vi "Acoustic modem TCPIP.vi"(2 "strings num":i32, 6 "Enum":T1(ring)=enum."bitrate", 7 "lOPP COUNT":i32, 8 "error in (no error)":errorcluster, 10 "Read/Write":bool, 11 "Cluster":T2) -> (0 "error out":errorcluster, 4 "Data Tx/Rx":string, 5 "Data out":string)   [LabVIEW 2021]
uses:
  183c8938-68d7-426e-a12b-0680b4555289.vi
panel:
  in  "error out 2":errorcluster
  out "x-y":u32
  out "WRITE BUTTON":bool
  in  "Write Power Status":bool
  out "match substring":string
  out "Modem Ready Status":bool
  out "length":i32
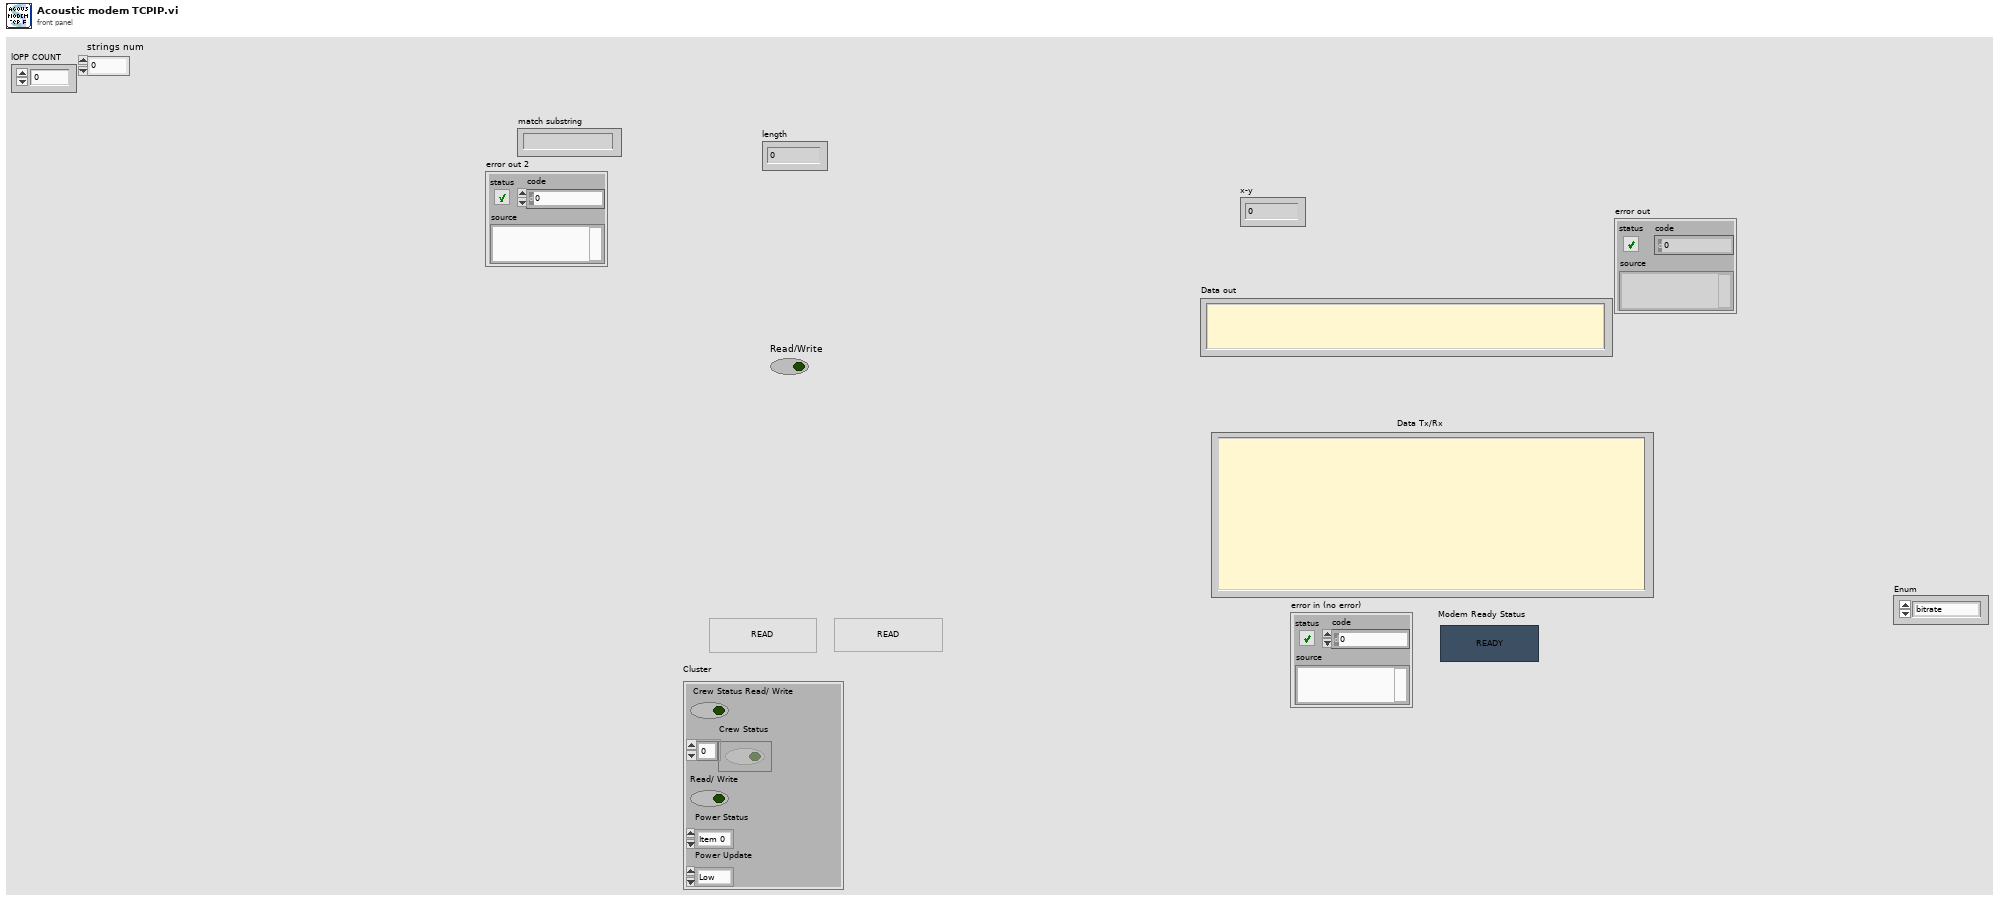
[diagram p1: front panel]
types:
  T1 = enum16{"TCPIP acoustic stop", "read write state", "command mode", "Disable Extended Notification", "bitrate", "initialization", "Int Power Status"}
  T2 = cluster{" Crew Status Read/ Write":bool, "Crew Status":bool[], "Read/ Write":bool, "Power Status":enum32{"Item 0", "Item 1", "Item 2", "Item 3"}, "Power Update":enum16{"Low", "Medium", "High", "Very High"}}
  T3 = cluster{"navigation":string, "HSSS":string, "P1":string, "P2":string}
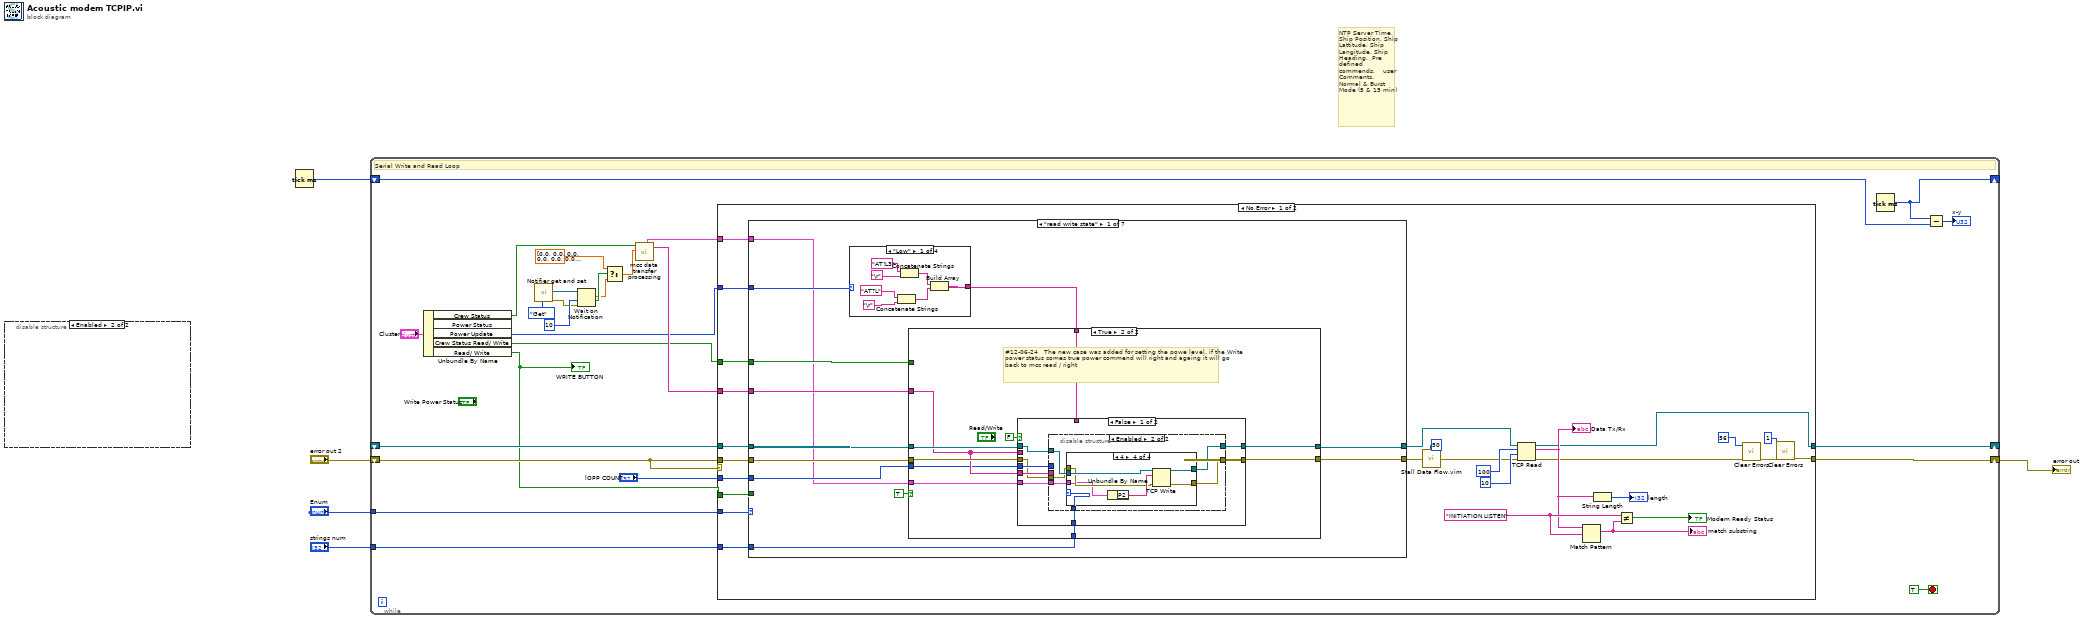
[diagram p0: block diagram]
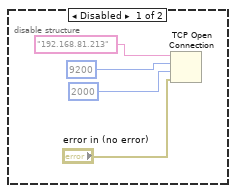
[diagram p2: hidden frame]
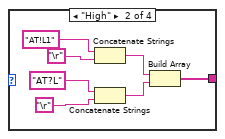
[diagram p3: hidden frame]
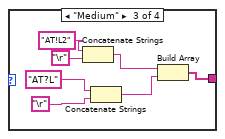
[diagram p4: hidden frame]
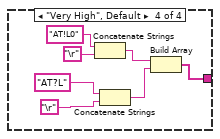
[diagram p5: hidden frame]
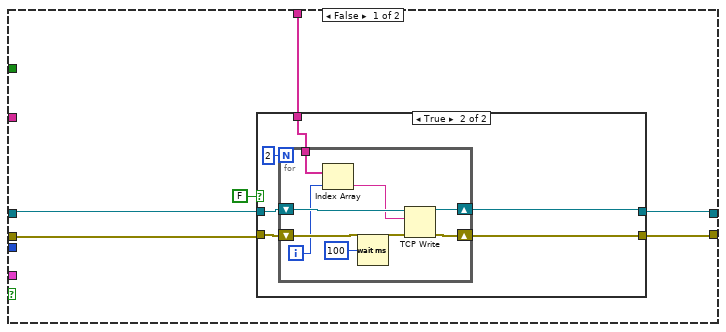
[diagram p6: hidden frame]
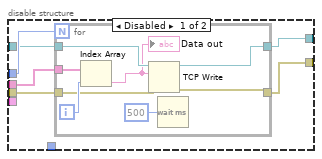
[diagram p8: hidden frame]
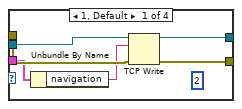
[diagram p9: hidden frame]
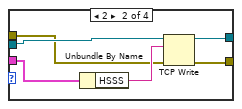
[diagram p10: hidden frame]
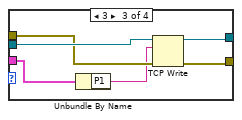
[diagram p11: hidden frame]
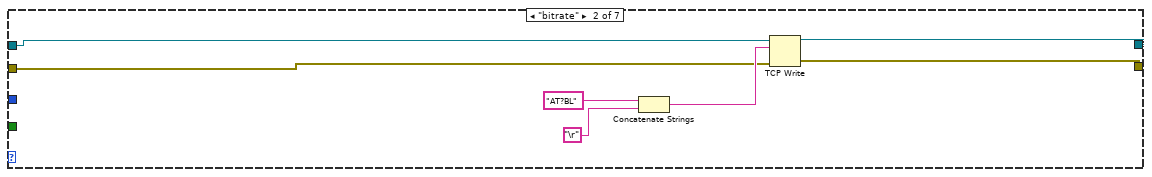
[diagram p13: hidden frame]
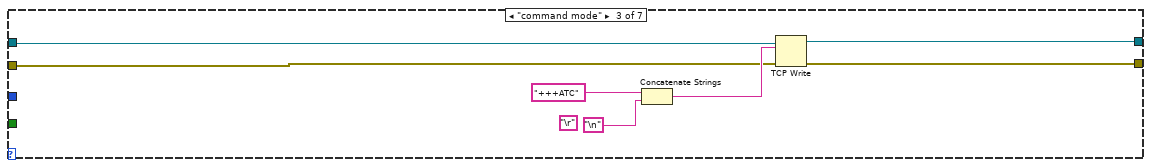
[diagram p14: hidden frame]
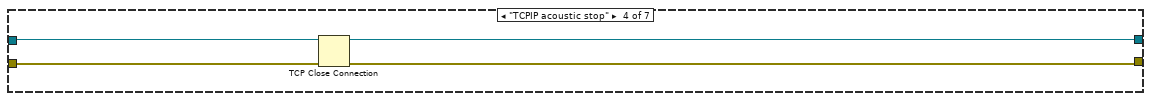
[diagram p15: hidden frame]
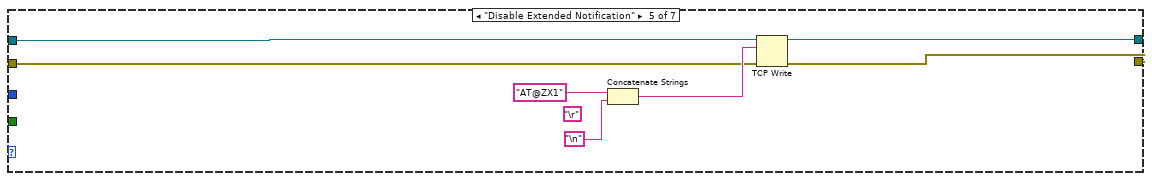
[diagram p16: hidden frame]
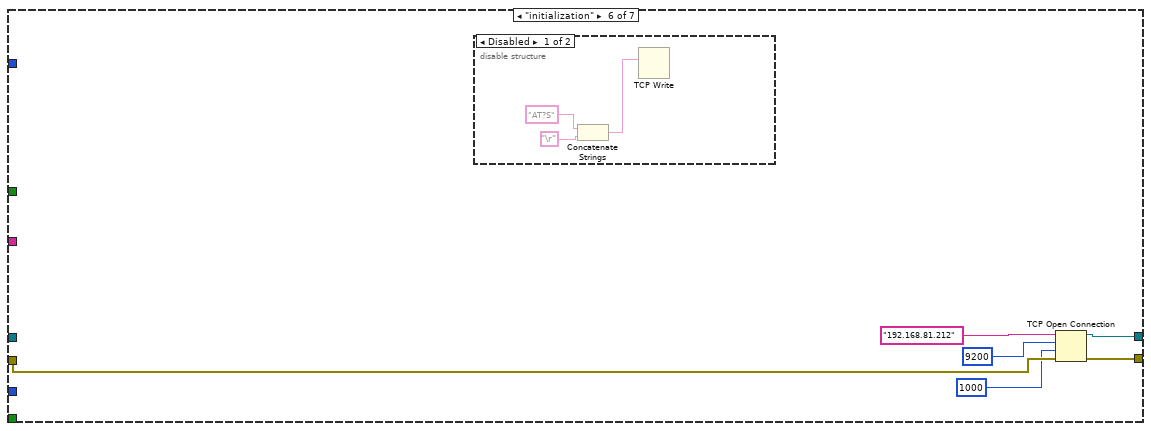
[diagram p17: hidden frame]
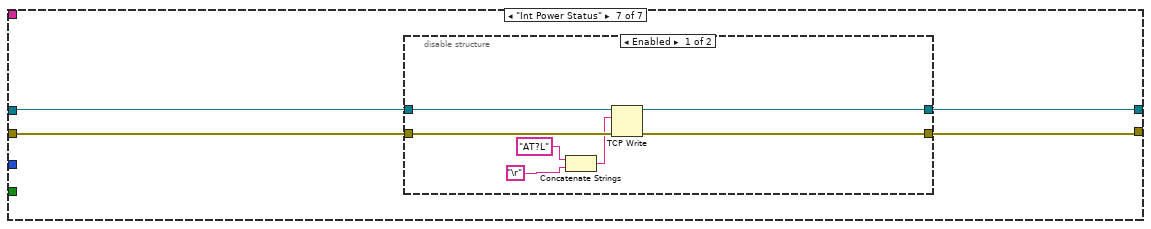
[diagram p19: hidden frame]
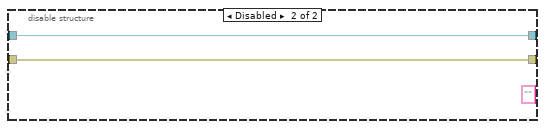
[diagram p20: hidden frame]
diagram:
  # "NTP Server Time, Ship Position, Ship Lattitude, Ship Langitude, Ship Heading,  Pre defined commends,    user Comments.  Normal & Burst Mode (5 & 15 min)"
  n1 = disable-structure shown="Enabled" {
    frame Disabled {
      n2 = TCP Open Connection(address="192.168.81.213", remote port or service name=u16 9200, timeout ms (60000)=2000, error in (no error)="error in (no error)") -> ()  [unwired: 1 in, 2 out]
    }
    frame Enabled {
    }
  }
  n3 = Tick Count (ms)() -> (millisecond timer value=w4:u32)
  n4 = while {
    shift-right: [w32] -> _
    shift-left: _ -> [w35]
    shift-right: [w31] -> w3
    shift-left: "error out 2" -> [w34]
    tunnel: "Enum" -> [w33]
    shift-right: [w14] -> _
    shift-left: w4 -> [w13]
    tunnel: "strings num" -> [w12]
    stop <- TRUE stop-if-true
    # "Serial Write and Read Loop"
    n5 = Unbundle By Name("Cluster") -> ("Crew Status"=w27:bool[], "Power Update"=w26:enum16{"Low", "Medium", "High", "Very High"}, "Crew Status Read/ Write"=w25:bool, "Read/ Write"=w24:bool)  [unwired: 1 out]
    "WRITE BUTTON" <- w24
    n6 = call "Notifier get and set.vi"("Operation"=enum16{"Init", "Get", "Set"}."Get") -> ("error out"=w18:errorcluster, "notifier out"=w21:refnum<notifier>)  [unwired: 9 in]
    n7 = Wait on Notification(notifier=w21, timeout in ms (-1)=10, error in (no error)=w18) -> (notification=w16:dbl[], timed out?=w17:bool)  [unwired: 1 in, 2 out]
    n8 = Select(t=dbl[] [0.0, 0.0, 0.0, 0.0, 0.0, 0.0, 0.0, 0.0, 0.0, 0.0, 0.0, 0.0, 0.0, 0.0, 0.0, 0.0, 0.0, 0.0, 0.0, 0.0, 0.0, 0.0, 0.0, 0.0, 0.0, 0.0, 0.0, 0.0, 0.0, 0.0, 0.0, 0.0, 0.0, 0.0, 0.0, 0.0, 0.0, 0.0, 0.0, 0.0, 0.0, 0.0, 0.0, 0.0, 0.0, 0.0, 0.0, 0.0, 0.0, 0.0, 0.0], s=w17, f=w16) -> (s? t:f=w22:dbl[])
    n9 = call "mcc data transfer processing.vi"("s? t:f"=w22, "Crew Status"=w27) -> ("output cluster"=w11:T3, "appended array"=w30:string[])  [unwired: 3 in, 4 out]
    n10 = case shown="No Error" w34 {
      selector: w34 -> [_ w238]
      tunnel: w35 -> [w62 _]
      tunnel: w34 -> [w61 _]
      tunnel: [w39 w242] -> w32
      tunnel: [w40 w241] -> w31
      tunnel: w24 -> [w57 _]
      tunnel: w33 -> [w54 _]
      tunnel: w30 -> [w53 _]
      tunnel: w25 -> [w51 _]
      tunnel: w26 -> [w49 _]
      tunnel: "lOPP COUNT" -> [w48 _]
      tunnel: w12 -> [w37 _]
      tunnel: w11 -> [w36 _]
      frame No Error {
        w60 = "INITIATION LISTEN"
        n11 = case shown="\"read write state\"" w54 {
          tunnel: w62 -> [w74 w189 w200 w206 w211 _ w225]
          tunnel: w61 -> [w73 w190 w199 w205 w210 w217 w226]
          tunnel: [w72 w191 w198 w204 w209 w215 w224] -> w45
          tunnel: [w71 w192 w197 w203 w208 w214 w223] -> w52
          tunnel: w57 -> [_ _ _ _ _ _ _]
          tunnel: w53 -> [w70 _ _ _ _ _ _]
          tunnel: w51 -> [w68 _ _ _ _ _ _]
          tunnel: w49 -> [w67 _ _ _ _ _ _]
          tunnel: w48 -> [w66 _ _ _ _ _ _]
          tunnel: w37 -> [w64 _ _ _ _ _ _]
          tunnel: w36 -> [w63 _ _ _ _ _ _]
          frame "read write state" {
            n12 = case shown="\"Low\"" w67 {
              tunnel: [w75 w84 w91 w96] -> w69
              frame "Low" {
                n13 = Concatenate Strings("AT?L" ("write buffer"), "\r") -> (w76:string)
                n14 = Concatenate Strings("AT!L3" ("string"), "\r") -> (w77:string)
                n15 = Build Array(w77, w76) -> (w75:string[])
              }
              frame "High" {
                n16 = Concatenate Strings("AT!L1" ("string"), "\r") -> (w83:string)
                n17 = Concatenate Strings("AT?L" ("write buffer"), "\r") -> (w82:string)
                n18 = Build Array(w83, w82) -> (w84:string[])
              }
              frame "Medium" {
                n19 = Concatenate Strings("AT!L2" ("string"), "\r") -> (w90:string)
                n20 = Concatenate Strings("AT?L" ("write buffer"), "\r") -> (w89:string)
                n21 = Build Array(w90, w89) -> (w91:string[])
              }
              frame "Very High", Default {
                n22 = Concatenate Strings("AT!L0" ("string"), "\r") -> (w98:string)
                n23 = Concatenate Strings("AT?L" ("write buffer"), "\r") -> (w97:string)
                n24 = Build Array(w98, w97) -> (w96:string[])
              }
            }
            n25 = case shown="True" TRUE {
              tunnel: w74 -> [w106 w134]
              tunnel: w73 -> [w108 w133]
              tunnel: [w105 w132] -> w72
              tunnel: [w107 w131] -> w71
              tunnel: w70 -> [_ w129]
              tunnel: w69 -> [w104 w130]
              tunnel: w68 -> [_ _]
              tunnel: w66 -> [_ w128]
              tunnel: w64 -> [_ w127]
              tunnel: w63 -> [_ w126]
              frame False {
                n26 = case shown="True" FALSE {
                  tunnel: w106 -> [w110 w115]
                  tunnel: w108 -> [w109 w116]
                  tunnel: [w110 w112] -> w105
                  tunnel: [w109 w111] -> w107
                  tunnel: w104 -> [_ w114]
                  frame False {
                  }
                  frame True {
                    n27 = for {
                      N: 2 -> [_]
                      tunnel: w114 -> [w119]
                      shift-right: [w121] -> w111
                      shift-left: w116 -> [w124]
                      shift-right: [w122] -> w112
                      shift-left: w115 -> [w123]
                      i -> [w120]
                      n28 = Index Array(array=w119, index=w120) -> (element=w118:string)
                      n29 = Wait (ms)(milliseconds to wait=u32 100) -> ()  [unwired: 1 out]
                      n30 = TCP Write(connection ID=w123, data in=w118, error in (no error)=w124) -> (connection ID out=w122:refnum<k5>, error out=w121:errorcluster)  [unwired: 1 in, 1 out]
                    }
                  }
                }
              }
              frame True {
                # "#12-06-24   The new case was added for setting the powe level. if the Write power status comes true power commend will right and againg it will go back to mcc read / right"
                n31 = case shown="False" FALSE {
                  tunnel: w134 -> [w140 w188]
                  tunnel: w133 -> [w139 w187]
                  tunnel: [w138 w188] -> w132
                  tunnel: [w137 w187] -> w131
                  tunnel: w129 -> [_ _]
                  tunnel: w130 -> [_ _]
                  tunnel: w129 -> [w142 _]
                  tunnel: w128 -> [w141 _]
                  tunnel: w127 -> [w136 _]
                  tunnel: w126 -> [w135 _]
                  frame False {
                    n32 = disable-structure shown="Enabled" {
                      disable-tunnel: w142 -> [w148 _]
                      disable-tunnel: w141 -> [w147 _]
                      disable-tunnel: w140 -> [w146 w160]
                      disable-tunnel: w139 -> [w145 w159]
                      disable-tunnel: [w144 w158] -> w138
                      disable-tunnel: [w143 w157] -> w137
                      disable-tunnel: w136 -> [_ w162]
                      disable-tunnel: w135 -> [_ w161]
                      frame Disabled {
                        n33 = for {
                          N: w147 -> [_]
                          tunnel: w148 -> [w156]
                          tunnel: w146 -> [w154]
                          tunnel: [w152] -> w144
                          tunnel: w145 -> [w153]
                          tunnel: [w151] -> w143
                          i -> [w155]
                          n34 = Index Array(array=w156, index=w155) -> (element=w150:string)
                          "Data out" <- w150
                          n35 = TCP Write(connection ID=w154, data in=w150, error in (no error)=w153) -> (connection ID out=w152:refnum<k5>, error out=w151:errorcluster)  [unwired: 1 in, 1 out]
                          n36 = Wait (ms)(milliseconds to wait=u32 500) -> ()  [unwired: 1 out]
                        }
                      }
                      frame Enabled {
                        n37 = case shown="4" w162 {
                          tunnel: w161 -> [w166 w173 w175 w181]
                          tunnel: w160 -> [w168 w172 w178 w183]
                          tunnel: w159 -> [w167 w171 w177 w182]
                          tunnel: [w164 w170 w180 w184] -> w158
                          tunnel: [w163 w169 w179 w185] -> w157
                          frame 1, Default {
                            (unwired) 2
                            n38 = Unbundle By Name(w166) -> ("navigation"=w165:string)
                            n39 = TCP Write(connection ID=w168, data in=w165, error in (no error)=w167) -> (connection ID out=w164:refnum<k5>, error out=w163:errorcluster)  [unwired: 1 in, 1 out]
                          }
                          frame 2 {
                            n40 = Unbundle By Name(w173) -> ("HSSS"=w174:string)
                            n41 = TCP Write(connection ID=w172, data in=w174, error in (no error)=w171) -> (connection ID out=w170:refnum<k5>, error out=w169:errorcluster)  [unwired: 1 in, 1 out]
                          }
                          frame 3 {
                            n42 = Unbundle By Name(w175) -> ("P1"=w176:string)
                            n43 = TCP Write(connection ID=w178, data in=w176, error in (no error)=w177) -> (connection ID out=w180:refnum<k5>, error out=w179:errorcluster)  [unwired: 1 in, 1 out]
                          }
                          frame 4 {
                            n44 = Unbundle By Name(w181) -> ("P2"=w186:string)
                            n45 = TCP Write(connection ID=w183, data in=w186, error in (no error)=w182) -> (connection ID out=w184:refnum<k5>, error out=w185:errorcluster)  [unwired: 1 in, 1 out]
                          }
                        }
                      }
                    }
                  }
                  frame True {
                  }
                }
              }
            }
          }
          frame "bitrate" {
            n46 = Concatenate Strings("AT?BL" ("string"), "\r") -> (w195:string)
            n47 = TCP Write(connection ID=w189, data in=w195, error in (no error)=w190) -> (connection ID out=w191:refnum<k5>, error out=w192:errorcluster)  [unwired: 1 in, 1 out]
          }
          frame "command mode" {
            (unwired) "\r"
            n48 = Concatenate Strings("+++ATC" ("string"), "\n") -> (w201:string)
            n49 = TCP Write(connection ID=w200, data in=w201, error in (no error)=w199) -> (connection ID out=w198:refnum<k5>, error out=w197:errorcluster)  [unwired: 1 in, 1 out]
          }
          frame "TCPIP acoustic stop" {
            n50 = TCP Close Connection(connection ID=w206, error in (no error)=w205) -> (connection ID out=w204:refnum<k5>, error out=w203:errorcluster)  [unwired: 1 in]
          }
          frame "Disable Extended Notification" {
            (unwired) "\r"
            n51 = Concatenate Strings("AT@ZX1" ("string"), "\n") -> (w213:string)
            n52 = TCP Write(connection ID=w211, data in=w213, error in (no error)=w210) -> (connection ID out=w209:refnum<k5>, error out=w208:errorcluster)  [unwired: 1 in, 1 out]
          }
          frame "initialization" {
            n53 = disable-structure shown="Disabled" {
              frame Disabled {
                n54 = Concatenate Strings("AT?S" ("string"), "\r") -> (w222:string)
                n55 = TCP Write(data in=w222) -> ()  [unwired: 3 in, 3 out]
              }
              frame Enabled {
              }
            }
            n56 = TCP Open Connection(address="192.168.81.212", remote port or service name=u16 9200, timeout ms (60000)=1000, error in (no error)=w217) -> (connection ID=w215:refnum<k5>, error out=w214:errorcluster)  [unwired: 1 in]
          }
          frame "Int Power Status" {
            n57 = disable-structure shown="Enabled" {
              disable-tunnel: w226 -> [w233 w235]
              disable-tunnel: w225 -> [w232 w236]
              disable-tunnel: [w227 w236] -> w224
              disable-tunnel: [w228 w235] -> w223
              frame Enabled {
                n58 = Concatenate Strings("AT?L" ("write buffer"), "\r") -> (w230:string)
                n59 = TCP Write(connection ID=w232, data in=w230, error in (no error)=w233) -> (connection ID out=w227:refnum<k5>, error out=w228:errorcluster)  [unwired: 1 in, 1 out]
              }
              frame Disabled {
                w234 = "" ("read buffer")
              }
            }
          }
        }
        n60 = call "Stall Data Flow.vim"("value in"=w52, "milliseconds to wait"=u32 50) -> ("value out"=w44:errorcluster)  [unwired: 1 out]
        n61 = TCP Read(connection ID=w45, bytes to read=100, error in (no error)=w44, 9:10 ("timeout ms (25000)")) -> (connection ID out=w39:refnum<k5>, data out=w56:string, error out=w43:errorcluster)  [unwired: 1 in]
        "Data Tx/Rx" <- w56
        n62 = Match Pattern(string=w56, regular expression=w60) -> (match substring=w59:string)  [unwired: 1 in, 3 out]
        "match substring" <- w59
        n63 = String Length(string=w56) -> (length=→"length":i32)
        n64 = Not Equal?(x=w60, y=w59) -> (x != y?=→"Modem Ready Status":bool)
        n65 = call <vilib>:"Clear Errors.vi"("error in (no error)"=w43, "specific error code to clear (0: all)"=56) -> ("error out"=w38:errorcluster)  [unwired: 4 in, 1 out]
        n66 = call <vilib>:"Clear Errors.vi"("error in (no error)"=w38, "specific error code to clear (0: all)"=1) -> ("error out"=w40:errorcluster)  [unwired: 4 in, 1 out]
      }
      frame Error {
        n67 = call <vilib>:"Clear Errors.vi"("error in (no error)"=w238) -> ("error out"=w237:errorcluster)  [unwired: 5 in, 1 out]
        n68 = flat-sequence {
          tunnel: [w243] -> w239
          tunnel: w237 -> [w243]
          tunnel: [w245] -> w240
          tunnel: w239 -> [w245]
          tunnel: [w250] -> w242
          tunnel: [w249] -> w241
          tunnel: w240 -> [w248]
          frame #0 {
            n69 = Wait (ms)(milliseconds to wait=u32 100) -> ()  [unwired: 1 out]
          }
          frame #1 {
            n70 = Wait (ms)(milliseconds to wait=u32 100) -> ()  [unwired: 1 out]
          }
          frame #2 {
            n71 = TCP Open Connection(address="192.168.81.212", remote port or service name=u16 9200, timeout ms (60000)=2000, error in (no error)=w248) -> (connection ID=w250:refnum<k5>, error out=w249:errorcluster)  [unwired: 1 in]
          }
        }
      }
    }
    n72 = Tick Count (ms)() -> (millisecond timer value=w14:u32)
    n73 = Subtract(x=w14, y=w13) -> (x-y=→"x-y":u32)
  }
  "error out" <- w3
